vi "Global.field.vi"() -> ()   [LabVIEW 2009]
panel:
  in  "Field":bool
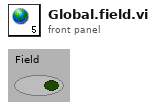
[diagram p1: front panel]
diagram:
